vi "Create.vi"(10 "Some Fancy Data":T1) -> (3 "ElementsValue out":refnum<class "ElementsValue.lvclass">)   [LabVIEW 2020, in "Futures-Examples.lvlib" / "ElementsValue.lvclass"]
uses:
  ElementsValue.lvclass
  Some Fancy Data.ctl
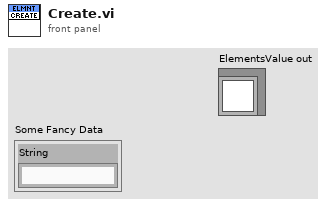
[diagram p1: front panel]
types:
  T1 = typedef "Futures-Examples.lvlib/ElementsValue.lvclass/Some Fancy Data.ctl" = cluster{"String":string}
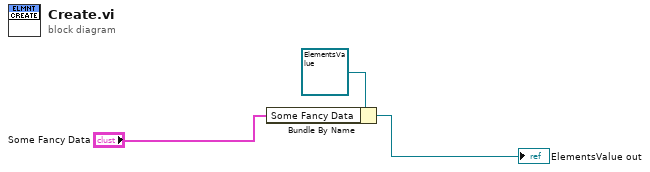
[diagram p0: block diagram]
diagram:
  n1 = Bundle By Name(cluster=refnum<class "ElementsValue.lvclass"> refnum ("ElementsValue in"), "Some Fancy Data"="Some Fancy Data") -> (→"ElementsValue out":refnum<class "ElementsValue.lvclass">)
